vi "Self-Test.vi"(8 "error in (no error)":errorcluster, 11 "VISA resource name":refnum<visa-resource-name>) -> (0 "error out":errorcluster, 1 "Self-Test Result Message":string, 2 "Self-Test Result Code":i32, 3 "VISA resource name out":refnum<visa-resource-name>)   [LabVIEW 2025, in "NewtonsPSM1735.lvlib"]
doc: "Runs the instrument's self-test routine and returns the test results.\nThe result should be 1."
uses:
  NewtonsPSM1735.lvlib
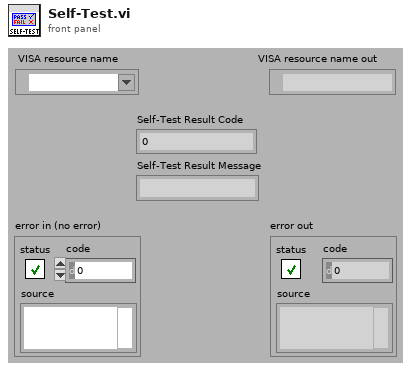
[diagram p1: front panel]
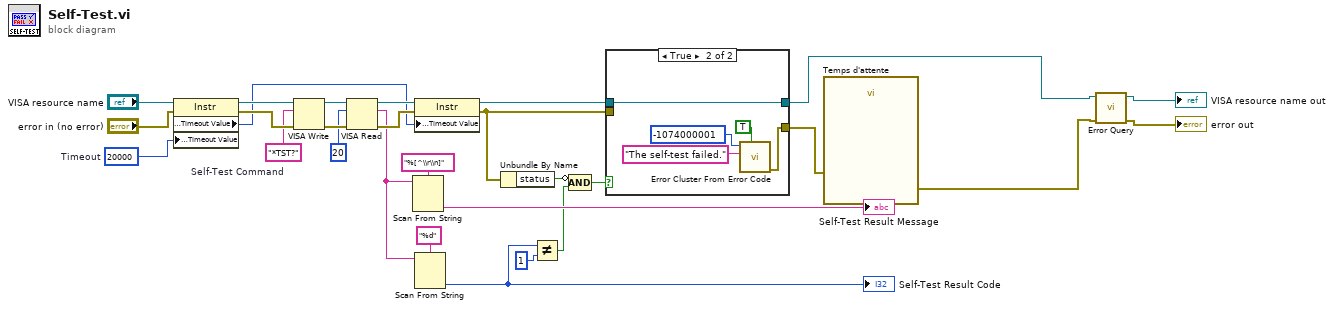
[diagram p0: block diagram]
diagram:
  w17 = u32 20000  # Timeout
  w13 = "*TST?"  # Self-Test Command
  n1 = property class="Instr"(reference="VISA resource name", error in="error in (no error)", "General Settings:Timeout Value"=w17) -> (reference out=w15:refnum<visa-resource-name>, error out=w16:errorcluster, "General Settings:Timeout Value"=w14:u32)
  n2 = VISA Write(VISA resource name=w15, write buffer=w13, error in (no error)=w16) -> (VISA resource name out=w24:refnum<visa-resource-name>, error out=w23:errorcluster)  [unwired: 1 out]
  n3 = VISA Read(VISA resource name=w24, byte count=u32 20 ("byte count (20)"), error in (no error)=w23) -> (VISA resource name out=w26:refnum<visa-resource-name>, read buffer=w19:string, error out=w25:errorcluster)  [unwired: 1 out]
  n4 = Scan From String(format string="%[^\\r\\n]" ("Format String"), input string=w19) -> (output 1=→"Self-Test Result Message":string)  [unwired: 2 in, 4 out]
  n5 = property class="Instr"(reference=w26, error in=w25, "General Settings:Timeout Value"=w14) -> (reference out=w12:refnum<visa-resource-name>, error out=w11:errorcluster)
  n6 = Scan From String(format string="%d", input string=w19) -> (output 1=w6:i32)  [unwired: 2 in, 4 out]
  "Self-Test Result Code" <- w6
  n7 = Unbundle By Name(w11) -> ("status"=w8:bool)
  n8 = Not Equal?(x=w6, y=1) -> (x != y?=w9:bool)
  n9 = Compound Arithmetic op=AND(invert w8, w9) -> (w7:bool)
  n10 = case shown="True" w7 {
    tunnel: w12 -> [w30 w35]
    tunnel: w11 -> [w29 _]
    tunnel: [w29 w31] -> w10
    tunnel: [w30 w35] -> w1
    frame False {
    }
    frame True {
      n11 = call <vilib>:"Error Cluster From Error Code.vi"("show call chain? (False)"=TRUE, "error message (\"\")"="The self-test failed." ("Source (VI Name)"), "error code (0)"=-1074000001 ("Code")) -> ("error out"=w31:errorcluster)  [unwired: 1 in, 5 out]
    }
  }
  n12 = call "Temps d'attente"("error in (no error)"=w10) -> ("error out"=w2:errorcluster)  [unwired: 1 in, 9 out]
  n13 = call "Error Query.vi"("error in (no error)"=w2, "VISA resource name"=w1) -> ("error out"=→"error out":errorcluster, "VISA resource name out"=→"VISA resource name out":refnum<visa-resource-name>)  [unwired: 8 out]
